vi "Easy XML Editor.vi"() -> ()   [LabVIEW 2023]
doc: "A tool for editing LabVIEW objects as XML that's quicker than using the other resource editor VI."
uses:
  CTLs/XML Editor State Data.ctl
  Resource Manipulation/Resource Array.ctl
  Resource Manipulation/Resource.ctl
  Resource Manipulation/Find Resource by Type (String).vi
  Resource Manipulation.lvlib
panel:
  in  "Paste FP":bool
  in  "Copy FP":bool
  in  "Front Panel XML/VTT":string
  in  "Paste BD":bool
  in  "Copy BD":bool
  in  "Block Diagram XML/VTT":string
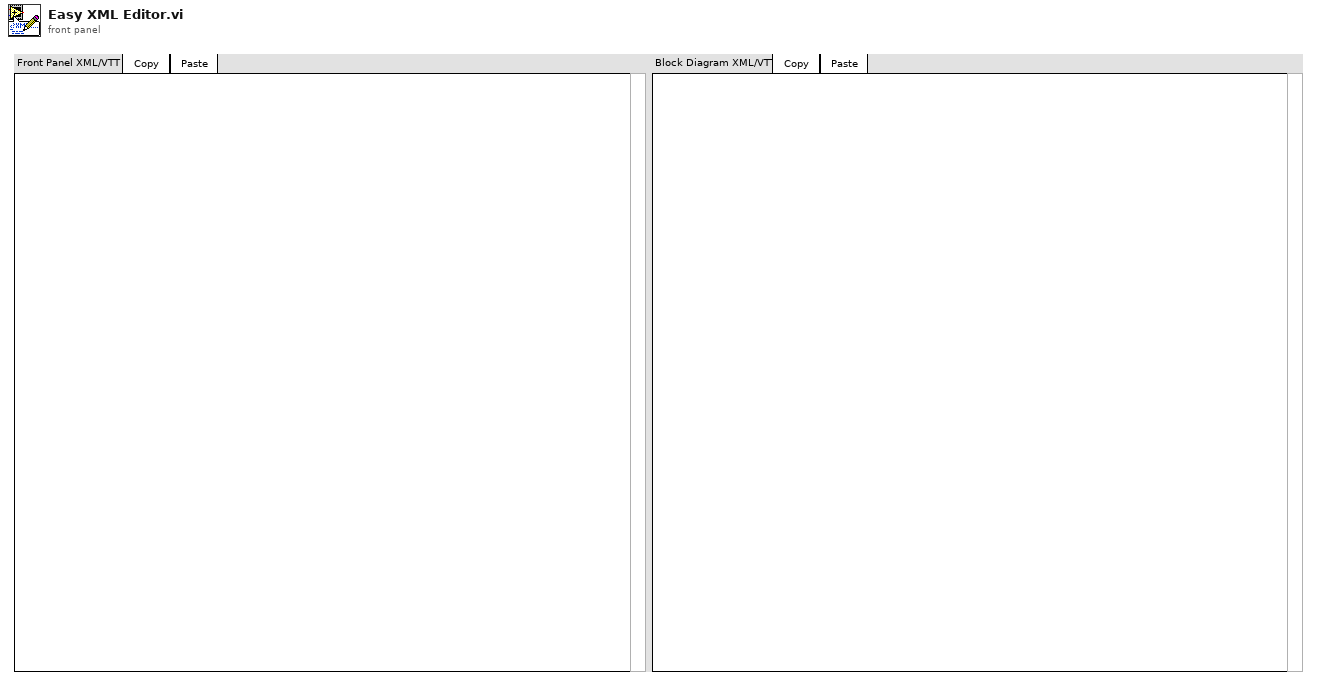
[diagram p1: front panel]
types:
  T1 = typedef "XML Editor State Data.ctl" = cluster{"Stored Resources":T2, "Use Stored Resources?":bool, "Last Edited VI Path":path, "Use VTT?":bool}
  T2 = typedef "Resource Manipulation.lvlib/Resource Array.ctl" = T3[]
  T3 = typedef "Resource Manipulation.lvlib/Resource.ctl" = cluster{"type":u32, "id":i32, "name":string, "binary data":string}
  T4 = typedef "LVPositionTypeDef.ctl" = cluster{"Left":i32, "Top":i32}
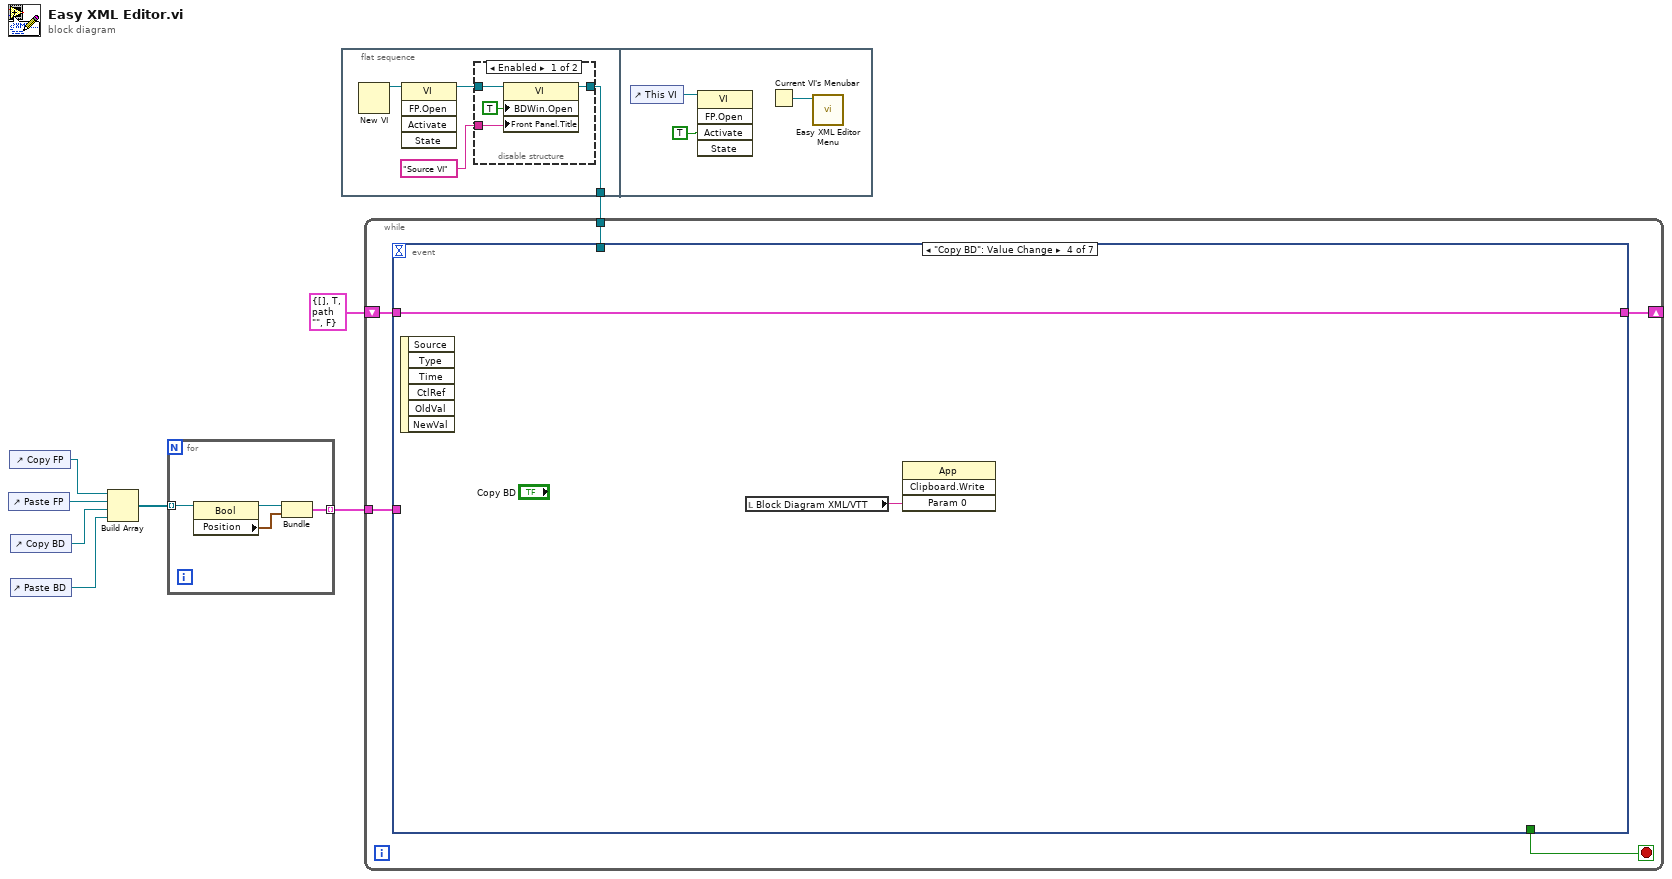
[diagram p0: block diagram]
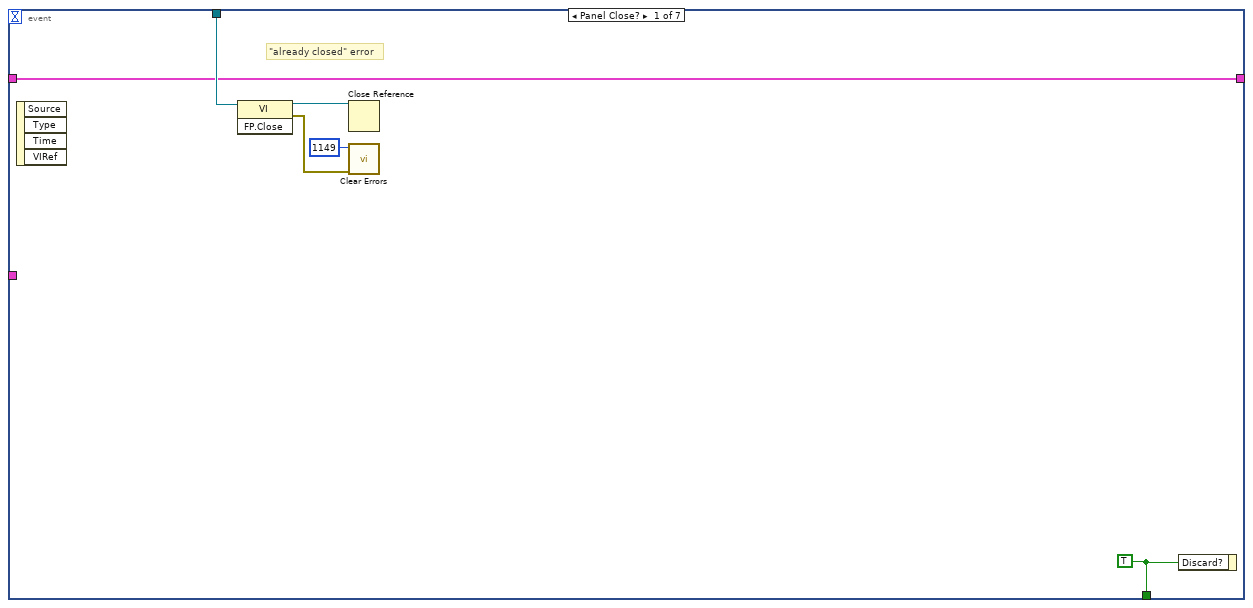
[diagram p2: hidden frame]
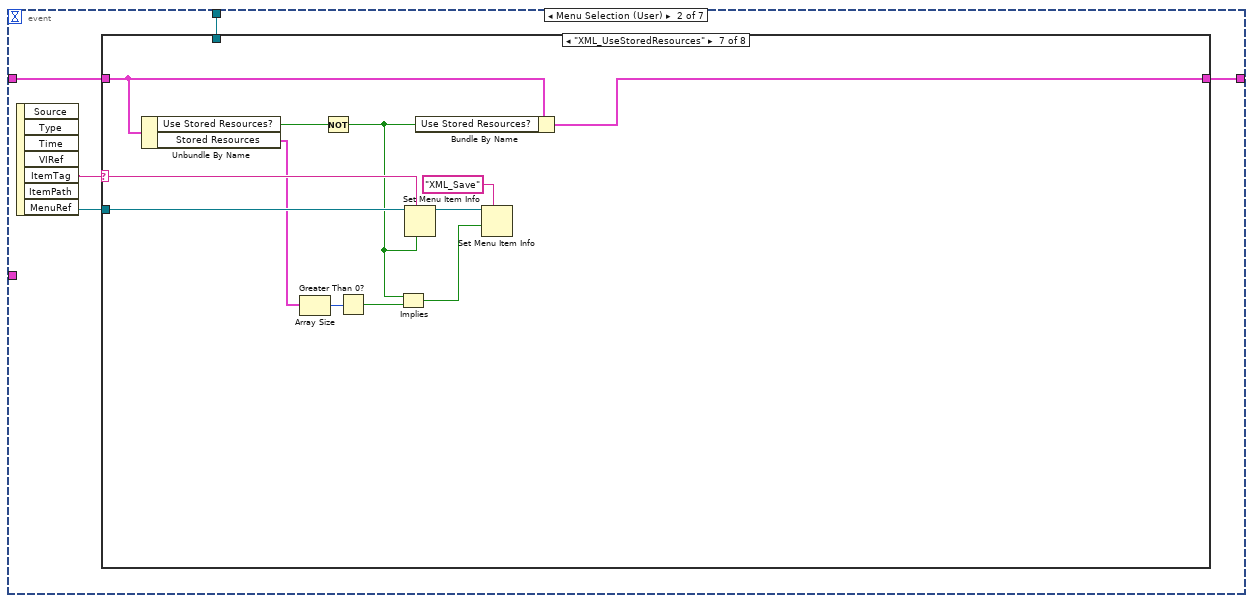
[diagram p3: hidden frame]
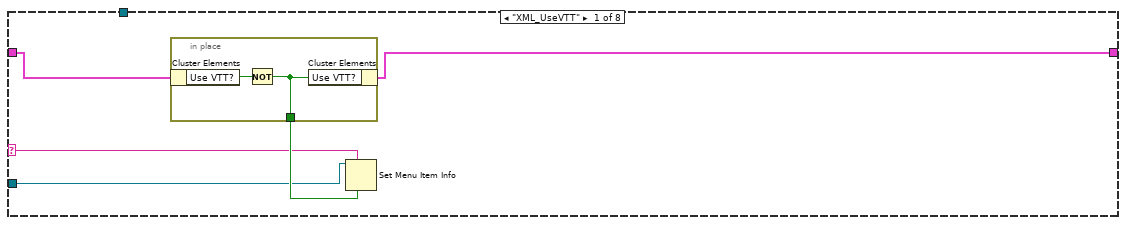
[diagram p4: hidden frame]
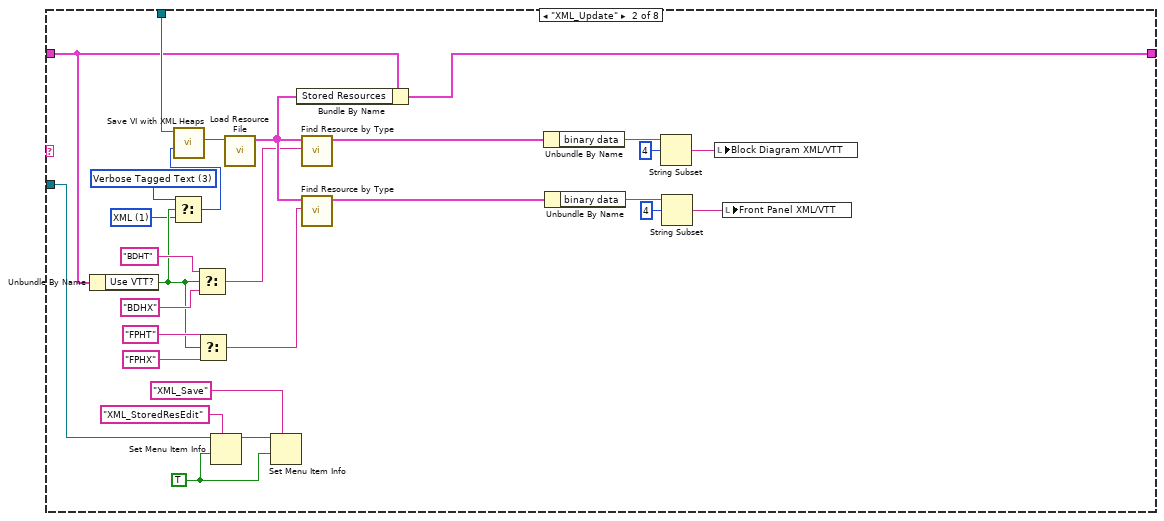
[diagram p5: hidden frame]
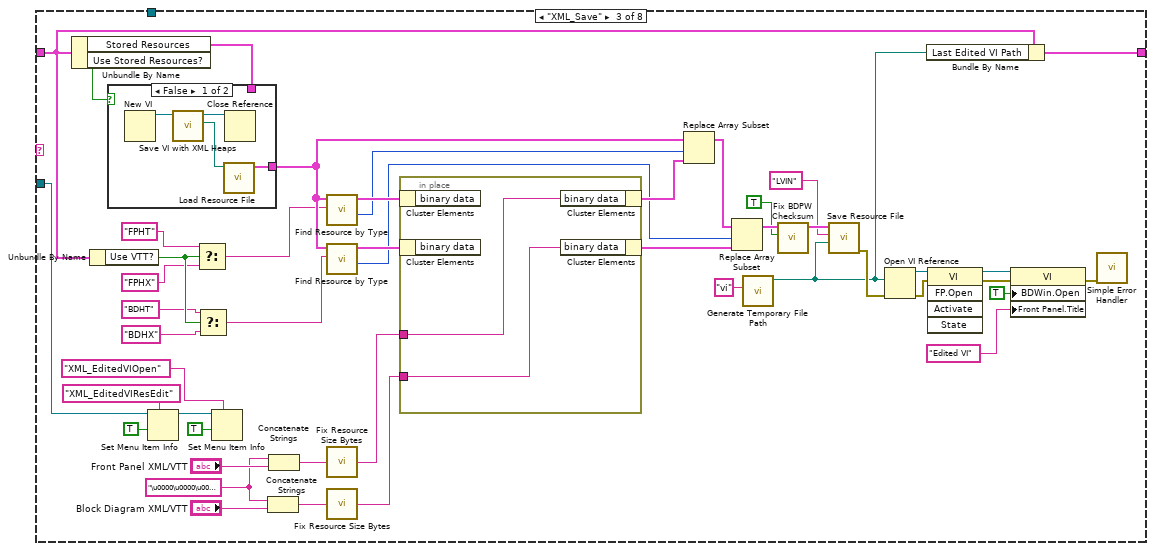
[diagram p6: hidden frame]
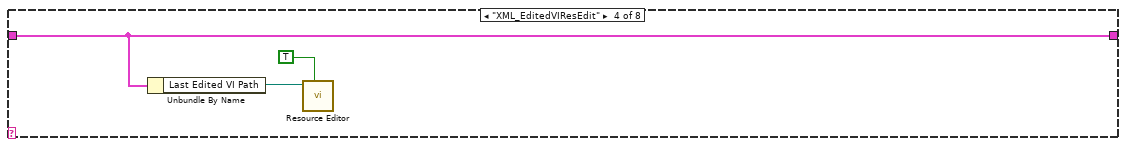
[diagram p8: hidden frame]
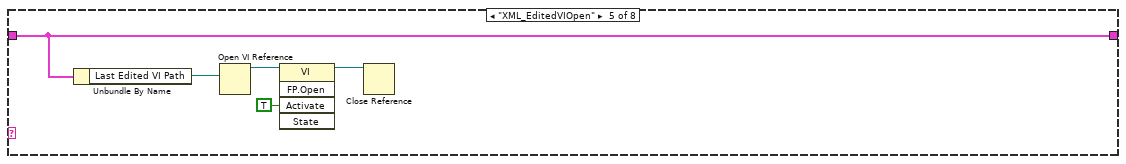
[diagram p9: hidden frame]
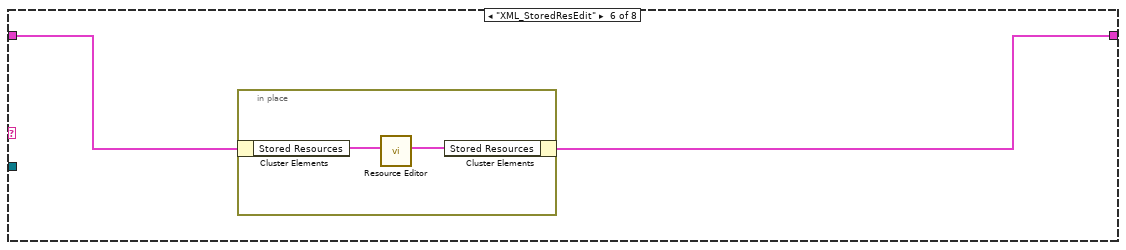
[diagram p10: hidden frame]
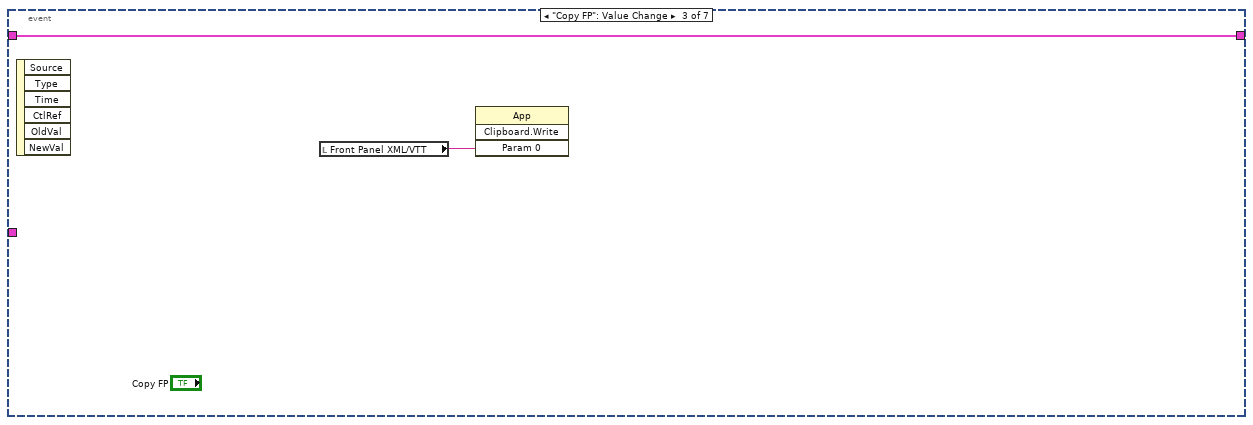
[diagram p12: hidden frame]
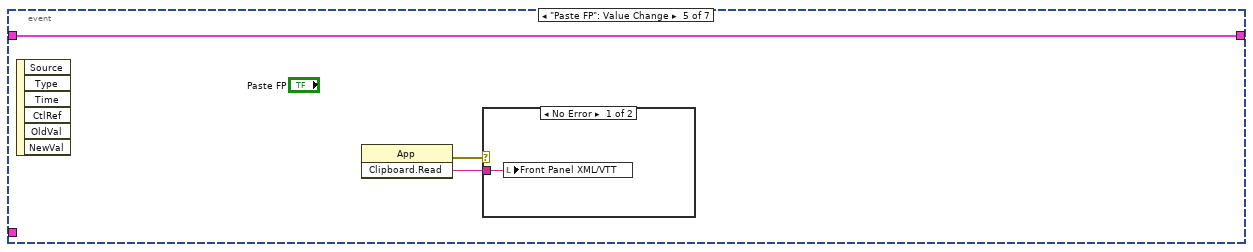
[diagram p13: hidden frame]
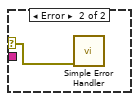
[diagram p14: hidden frame]
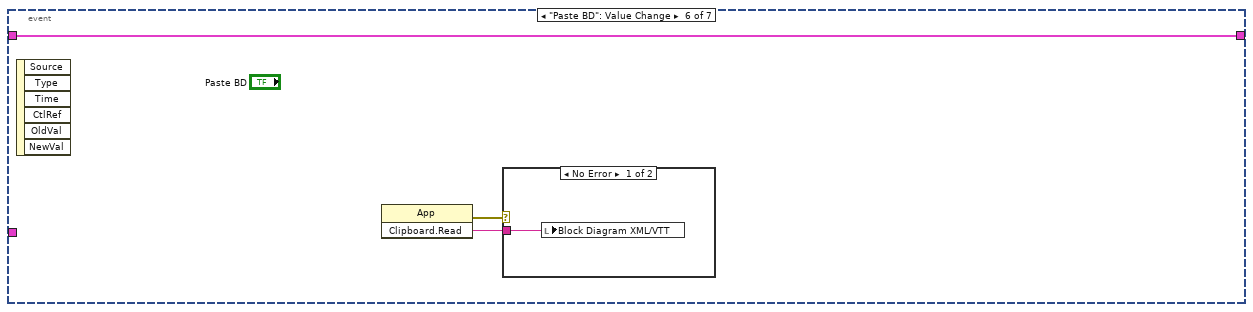
[diagram p15: hidden frame]
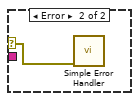
[diagram p16: hidden frame]
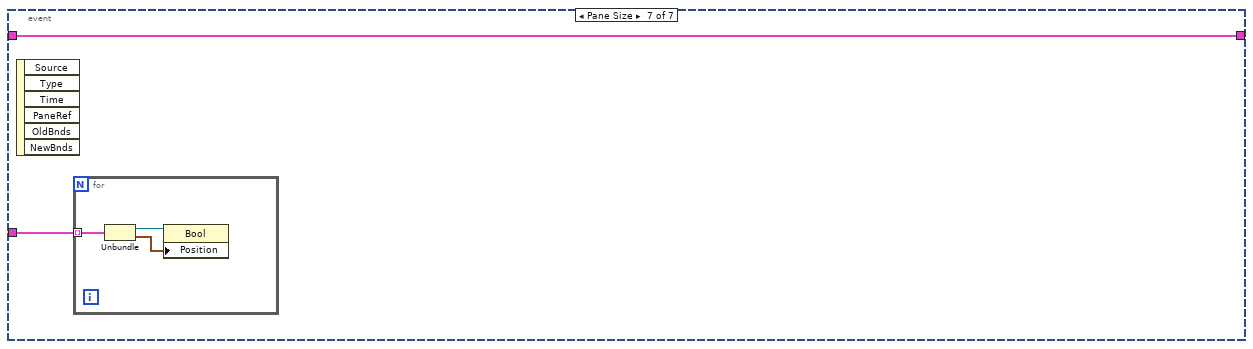
[diagram p17: hidden frame]
diagram:
  n1 = control-ref of="Paste FP"() -> (w5:refnum<vi>)
  n2 = control-ref of="Copy FP"() -> (w6:refnum<vi>)
  n3 = control-ref of="Copy BD"() -> (w4:refnum<vi>)
  n4 = control-ref of="Paste BD"() -> (w3:refnum<vi>)
  n5 = Build Array(w6, w5, w4, w3) -> (w2:refnum<vi>[])
  n6 = for {
    tunnel: w2 -> [w12] mode=indexing
    tunnel: [w9] -> w1 mode=indexing
    n7 = property class="Bool"(reference=w12) -> (reference out=w11:refnum<vi>, "Position"=w10:T4)  [unwired: 1 in, 1 out]
    n8 = Bundle("Paste BD"=w11, "Position"=w10) -> (w9:cluster{"Paste BD":refnum<vi>, "Position":T4})  [unwired: 1 in]
  }
  n9 = flat-sequence {
    tunnel: [w14] -> w8
    frame #0 {
      n10 = New VI() -> (3:w16:refnum<vi>)  [unwired: 7 in, 1 out]
      n11 = invoke class="VI" method="FP.Open"(reference=w16) -> (reference out=w15:refnum<vi>)  [unwired: 4 in, 4 out]
      n12 = disable-structure shown="Enabled" {
        disable-tunnel: w15 -> [w20 w21]
        disable-tunnel: [w18 w21] -> w14
        disable-tunnel: "Source VI" -> [w17 _]
        frame Enabled {
          n13 = property class="VI"(reference=w20, "BDWin.Open"=TRUE ("Block Diagram Window:Open"), "Front Panel.Title"=w17) -> (reference out=w18:refnum<vi>)  [unwired: 1 in, 1 out]
        }
        frame Disabled {
        }
      }
    }
    frame #1 {
      n14 = control-ref of="This VI"() -> (w24:refnum<vi>)
      n15 = invoke class="VI" method="FP.Open"(reference=w24, "Activate"=TRUE ("Activate?")) -> ()  [unwired: 3 in, 5 out]
      n16 = Current VI's Menubar() -> (w22:refnum<k9>)
      n17 = call "Easy XML Editor Menu.vi"("Menu Refnum In"=w22) -> ()  [unwired: 9 in, 2 out]
    }
  }
  n18 = while {
    tunnel: w8 -> [w29]
    shift-right: [w26] -> _
    shift-left: T1 {"Stored Resources"=[], "Use Stored Resources?"=TRUE, "Last Edited VI Path"=path "", "Use VTT?"=FALSE} ("Persistent State") -> [w27]
    tunnel: w1 -> [w25]
    stop <- w28 stop-if-true
    n19 = event shown="[3] \"Copy BD\": Value Change" {
      selector: _ -> [_ _ _ _ _ _ _]
      dyn-events: _ -> [_ _ _ _ _ _ _]
      timeout: _ -> [_ _ _ _ _ _ _]
      tunnel: w29 -> [w35 w39 _ _ _ _ _]
      tunnel: [w33 _ _ _ _ _ _] -> w28
      tunnel: w27 -> [w30 w38 w154 w156 w158 w163 w168]
      tunnel: [w30 w37 w154 w156 w158 w163 w168] -> w26
      tunnel: w25 -> [_ _ _ _ _ _ w169]
      event Panel Close? {
        w33 = TRUE
        # "\"already closed\" error"
        n20 = event-data() -> ()  [unwired: 1 in, 4 out]
        n21 = invoke class="VI" method="FP.Close"(reference=w35) -> (reference out=w34:refnum<vi>, error out=w32:errorcluster)  [unwired: 2 in, 1 out]
        n22 = Close Reference(reference=w34) -> ()  [unwired: 1 in, 1 out]
        n23 = call <vilib>:"Clear Errors.vi"("error in (no error)"=w32, "specific error code to clear (0: all)"=1149) -> ()  [unwired: 4 in, 2 out]
        n24 = event-data("Discard?"=w33) -> ()  [unwired: 1 in, 1 out]
      }
      event Menu Selection (User) {
        n25 = event-data() -> ("ItemTag"=w40:string, "MenuRef"=w36:refnum<k9>)  [unwired: 1 in, 5 out]
        n26 = case shown="\"XML_UseStoredResources\"" w40 {
          selector: w40 -> [w43 _ _ _ _ _ w148 _]
          tunnel: w39 -> [_ w75 _ _ _ _ _ _]
          tunnel: w38 -> [w45 w59 w76 w131 w136 w138 w151 w153]
          tunnel: [w42 w64 w91 w131 w136 w137 w150 w153] -> w37
          tunnel: w36 -> [w41 w63 w89 _ _ _ w149 _]
          frame "XML_UseVTT" {
            n27 = in-place {
              in-place-border: [w46] -> w44
              n28 = in-place-cluster #1(w45) -> ("Use VTT?"=w47:bool)
              n29 = Not(x=w47) -> (.not. x?=w46:bool)
              n30 = in-place-cluster #1("Use VTT?"=w46) -> (w42:T1)
            }
            n31 = Set Menu Item Info(6:w44, 7:w43, 11:w41) -> ()  [unwired: 4 in, 2 out]
          }
          frame "XML_Update" {
            w50 = u16 3 items=["Off", "XML", "Binary", "Verbose Tagged Text", "Binary2"] ("Heap Save Format (1=XML)")
            w49 = u16 1 items=["Off", "XML", "Binary", "Verbose Tagged Text", "Binary2"] ("Heap Save Format (1=XML)")
            w60 = TRUE ("enabled")
            n32 = Unbundle By Name(w59) -> ("Use VTT?"=w51:bool)
            n33 = Select(t=w50, s=w51, f=w49) -> (s? t:f=w48:u16)
            n34 = call "Save VI with XML Heaps.vi"("Heap Save Format (1=XML)"=w48, "VI Refnum In"=w75) -> ("VI Path out"=w74:path)  [unwired: 7 in, 2 out]
            n35 = Select(t="BDHT", s=w51, f="BDHX") -> (s? t:f=w53:string)
            n36 = Select(t="FPHT", s=w51, f="FPHX") -> (s? t:f=w52:string)
            n37 = Set Menu Item Info(7:"XML_StoredResEdit", 9:w60, 11:w63) -> (3:w61:refnum<k9>)  [unwired: 4 in, 1 out]
            n38 = call "Load Resource File.vi"("Resource File"=w74) -> ("Resources"=w65:T2)  [unwired: 8 in, 2 out]
            n39 = Set Menu Item Info(7:"XML_Save", 9:w60, 11:w61) -> ()  [unwired: 4 in, 2 out]
            n40 = Bundle By Name(cluster=w59, "Stored Resources"=w65) -> (w64:T1)
            n41 = call-poly "Find Resource by Type.vi"("Resource Type"=w53, "Resources"=w65) -> ("Resource"=w70:T3)  [unwired: 6 in, 3 out]
            n42 = call-poly "Find Resource by Type.vi"("Resource Type"=w52, "Resources"=w65) -> ("Resource"=w66:T3)  [unwired: 6 in, 3 out]
            n43 = Unbundle By Name(w70) -> ("binary data"=w73:string)
            n44 = Unbundle By Name(w66) -> ("binary data"=w67:string)
            n45 = String Subset(string=w73, offset (0)=4) -> (substring=w71:string)  [unwired: 1 in]
            n46 = String Subset(string=w67, offset (0)=4) -> (substring=w69:string)  [unwired: 1 in]
            n47 = local write "Block Diagram XML/VTT"(w71) -> ()
            n48 = local write "Front Panel XML/VTT"(w69) -> ()
          }
          frame "XML_Save" {
            w119 = "\u0000\u0000\u0000\u0000"
            n49 = Unbundle By Name(w76) -> ("Stored Resources"=w92:T2, "Use Stored Resources?"=w93:bool)
            n50 = Unbundle By Name(w76) -> ("Use VTT?"=w83:bool)
            n51 = case shown="False" w93 {
              tunnel: [w122 w126] -> w109
              tunnel: w92 -> [_ w126]
              frame False {
                n52 = New VI() -> (3:w125:refnum<vi>)  [unwired: 7 in, 1 out]
                n53 = call "Save VI with XML Heaps.vi"("VI Refnum In"=w125) -> ("VI Path out"=w123:path, "VI Refnum Out"=w124:refnum<vi>)  [unwired: 8 in, 1 out]
                n54 = call "Load Resource File.vi"("Resource File"=w123) -> ("Resources"=w122:T2)  [unwired: 8 in, 2 out]
                n55 = Close Reference(reference=w124) -> ()  [unwired: 1 in, 1 out]
              }
              frame True {
              }
            }
            n56 = Set Menu Item Info(7:"XML_EditedVIResEdit", 9:TRUE ("enabled"), 11:w89) -> (3:w86:refnum<k9>)  [unwired: 4 in, 1 out]
            n57 = Select(t="FPHT", s=w83, f="FPHX") -> (s? t:f=w78:string)
            n58 = Select(t="BDHT", s=w83, f="BDHX") -> (s? t:f=w77:string)
            n59 = Set Menu Item Info(7:"XML_EditedVIOpen", 9:TRUE ("enabled"), 11:w86) -> ()  [unwired: 4 in, 2 out]
            n60 = Concatenate Strings(w119, "Block Diagram XML/VTT") -> (w117:string)
            n61 = Concatenate Strings(w119, "Front Panel XML/VTT") -> (w118:string)
            n62 = call-poly "Find Resource by Type.vi"("Resource Type"=w78, "Resources"=w109) -> ("Index"=w112:i32, "Resource"=w114:T3)  [unwired: 6 in, 2 out]
            n63 = call-poly "Find Resource by Type.vi"("Resource Type"=w77, "Resources"=w109) -> ("Index"=w108:i32, "Resource"=w113:T3)  [unwired: 6 in, 2 out]
            n64 = call "Fix Resource Size Bytes.vi"("Data in"=w118) -> ("Data out"=w116:string)
            n65 = call "Fix Resource Size Bytes.vi"("Data in"=w117) -> ("Data out"=w115:string)
            n66 = in-place {
              in-place-border: w116 -> [w128]
              in-place-border: w115 -> [w127]
              n67 = in-place-cluster #2(w114) -> ()  [unwired: 1 out]
              n68 = in-place-cluster #3(w113) -> ()  [unwired: 1 out]
              n69 = in-place-cluster #2("binary data"=w128) -> (w111:T3)
              n70 = in-place-cluster #3("binary data"=w127) -> (w110:T3)
            }
            n71 = Replace Array Subset(array=w109, new element=w111, index=w112) -> (w107:T2)
            n72 = Replace Array Subset(array=w107, new element=w110, index=w108) -> (w100:T2)
            n73 = call <vilib>:"Generate Temporary File Path.vi"("Temporary File Extension (tmp)"="vi") -> ("Unique Temporary File Path"=w90:path)  [unwired: 9 in, 1 out]
            n74 = call "Fix BDPW Checksum.vi"("Only fix 3rd hash (F)"=TRUE, "Resources in"=w100) -> ("Resources out"=w99:T2)  [unwired: 9 in]
            n75 = call "Save Resource File.vi"("Path"=w90, "File type"="LVIN", "Resources"=w99) -> ("error out"=w105:errorcluster)  [unwired: 8 in]
            n76 = Open VI Reference(vi path=w90, error in (no error)=w105) -> (vi reference=w101:refnum<vi>, error out=w97:errorcluster)  [unwired: 4 in]
            n77 = Bundle By Name(cluster=w76, "Last Edited VI Path"=w90) -> (w91:T1)
            n78 = invoke class="VI" method="FP.Open"(reference=w101, error in=w97) -> (reference out=w102:refnum<vi>, error out=w96:errorcluster)  [unwired: 3 in, 3 out]
            n79 = property class="VI"(reference=w102, error in=w96, "BDWin.Open"=TRUE ("Block Diagram Window:Open"), "Front Panel.Title"="Edited VI") -> (error out=w95:errorcluster)  [unwired: 1 out]
            n80 = call <vilib>:"Simple Error Handler.vi"("error in (no error)"=w95) -> ()  [unwired: 4 in, 5 out]
          }
          frame "XML_EditedVIResEdit" {
            n81 = Unbundle By Name(w131) -> ("Last Edited VI Path"=w130:path)
            n82 = call "Resource Editor.vi"("Load from Initial Path (F)"=TRUE, "Path"=w130) -> ()  [unwired: 9 in, 1 out]
          }
          frame "XML_EditedVIOpen" {
            n83 = Unbundle By Name(w136) -> ("Last Edited VI Path"=w135:path)
            n84 = Open VI Reference(vi path=w135) -> (vi reference=w134:refnum<vi>)  [unwired: 5 in, 1 out]
            n85 = invoke class="VI" method="FP.Open"(reference=w134, "Activate"=TRUE ("Activate?")) -> (reference out=w132:refnum<vi>)  [unwired: 3 in, 4 out]
            n86 = Close Reference(reference=w132) -> ()  [unwired: 1 in, 1 out]
          }
          frame "XML_StoredResEdit" {
            n87 = in-place {
              n88 = in-place-cluster #4(w138) -> ("Stored Resources"=w140:T2)
              n89 = call "Resource Editor.vi"("Initial Resources"=w140) -> ("Final Resources"=w139:T2)  [unwired: 10 in]
              n90 = in-place-cluster #4("Stored Resources"=w139) -> (w137:T1)
            }
          }
          frame "XML_UseStoredResources" {
            n91 = Unbundle By Name(w151) -> ("Use Stored Resources?"=w152:bool, "Stored Resources"=w145:T2)
            n92 = Array Size(array=w145) -> (size(s)=w143:i32)
            n93 = Not(x=w152) -> (.not. x?=w144:bool)
            n94 = Greater Than 0?(x=w143) -> (x > 0?=w142:bool)
            n95 = Implies(1:w142, 2:w144) -> (0:w141:bool)
            n96 = Set Menu Item Info(6:w144, 7:w148, 11:w149) -> (3:w147:refnum<k9>)  [unwired: 4 in, 1 out]
            n97 = Bundle By Name(cluster=w151, "Use Stored Resources?"=w144) -> (w150:T1)
            n98 = Set Menu Item Info(7:"XML_Save" ("item tag"), 9:w141, 11:w147) -> ()  [unwired: 4 in, 2 out]
          }
          frame Default {
          }
        }
      }
      event "Copy FP": Value Change {
        n99 = event-data() -> ()  [unwired: 1 in, 6 out]
        n100 = local read "Front Panel XML/VTT"() -> (w155:string)
        n101 = invoke class="App" method="Clipboard.Write"("Param 0"=w155) -> ()  [unwired: 3 in, 4 out]
      }
      event "Copy BD": Value Change {
        n102 = event-data() -> ()  [unwired: 1 in, 6 out]
        n103 = local read "Block Diagram XML/VTT"() -> (w157:string)
        n104 = invoke class="App" method="Clipboard.Write"("Param 0"=w157) -> ()  [unwired: 3 in, 4 out]
      }
      event "Paste FP": Value Change {
        n105 = event-data() -> ()  [unwired: 1 in, 6 out]
        n106 = invoke class="App" method="Clipboard.Read"() -> (error out=w159:errorcluster, "Read Clipbrd"=w160:string)  [unwired: 3 in, 1 out]
        n107 = case shown="No Error" w159 {
          selector: w159 -> [_ w162]
          tunnel: w160 -> [w161 _]
          frame No Error {
            n108 = local write "Front Panel XML/VTT"(w161) -> ()
          }
          frame Error {
            n109 = call <vilib>:"Simple Error Handler.vi"("error in (no error)"=w162) -> ()  [unwired: 4 in, 5 out]
          }
        }
      }
      event "Paste BD": Value Change {
        n110 = event-data() -> ()  [unwired: 1 in, 6 out]
        n111 = invoke class="App" method="Clipboard.Read"() -> (error out=w164:errorcluster, "Read Clipbrd"=w165:string)  [unwired: 3 in, 1 out]
        n112 = case shown="No Error" w164 {
          selector: w164 -> [_ w167]
          tunnel: w165 -> [w166 _]
          frame No Error {
            n113 = local write "Block Diagram XML/VTT"(w166) -> ()
          }
          frame Error {
            n114 = call <vilib>:"Simple Error Handler.vi"("error in (no error)"=w167) -> ()  [unwired: 4 in, 5 out]
          }
        }
      }
      event Pane Size {
        n115 = event-data() -> ()  [unwired: 1 in, 6 out]
        n116 = for {
          tunnel: w169 -> [w172] mode=indexing
          n117 = Unbundle(w172) -> ("Paste BD"=w171:refnum<vi>, "Position"=w170:T4)
          n118 = property class="Bool"(reference=w171, "Position"=w170) -> ()  [unwired: 1 in, 2 out]
        }
      }
    }
  }
